vi "Close Panel.vi"(8 "error in (no error)":errorcluster, 10 "Panel":refnum<class "Panel.lvclass">, 11 "Manager in":refnum<class "Manager.lvclass">) -> (0 "error out":errorcluster, 3 "Manager out":refnum<class "Manager.lvclass">)   [LabVIEW 2020, in "OOPanel.lvlib" / "Manager.lvclass"]
uses:
  Manager.lvclass
  Manager.lvclass/Manager.ctl
  Panel/Panel.lvclass
  Panel/Close Reason.ctl
  OOPanel.lvlib
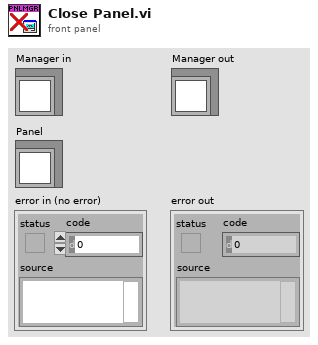
[diagram p1: front panel]
types:
  T1 = typedef "OOPanel.lvlib/Close Reason.ctl" = enum16{"Shutdown", "Close"}
  T2 = typedef "OOPanel.lvlib/Visibility State.ctl" = enum16{"Idle", "Closed", "Hidden", "Visible", "Subpanel"}
  T3 = typedef "OOPanel.lvlib/Manager.lvclass/Ref Data.ctl" = cluster{"SubPanel Map":T4, "Panels":refnum<class "Panel.lvclass">[]}
  T4 = typedef "OOPanel.lvlib/Manager.lvclass/SubPanel Map.ctl" = cluster{"SubPanels":refnum<vi>[], "Panels":refnum<class "Panel.lvclass">[]}
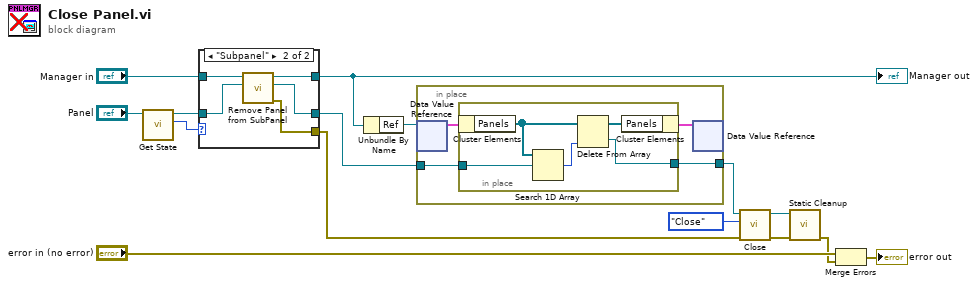
[diagram p0: block diagram]
diagram:
  n1 = call "Get State.vi"("Panel in"="Panel") -> ("State"=w13:T2, "Panel out"=w12:refnum<class "Panel.lvclass">)  [unwired: 8 in, 1 out]
  n2 = case shown="\"Subpanel\"" w13 {
    tunnel: w12 -> [w17 w21]
    tunnel: "Manager in" -> [w16 w22]
    tunnel: [w16 w20] -> w9
    tunnel: [w17 w19] -> w8
    tunnel: [_ w18] -> w7
    frame Default {
    }
    frame "Subpanel" {
      n3 = call "Remove Panel from SubPanel.vi"("Panel In"=w21, "Manager in"=w22) -> ("error out"=w18:errorcluster, "Panel"=w19:refnum<class "Panel.lvclass">, "Manager out"=w20:refnum<class "Manager.lvclass">)  [unwired: 7 in]
    }
  }
  "Manager out" <- w9
  n4 = Unbundle By Name(w9) -> ("Ref"=w10:refnum<data-value>)
  n5 = in-place {
    in-place-border: w8 -> [w24]
    in-place-border: [w23] -> w6
    n6 = in-place-dvr #1(w10) -> (w26:T3)  [unwired: 1 out]
    n7 = in-place {
      in-place-border: w24 -> [w31]
      in-place-border: [w27] -> w23
      n8 = in-place-cluster #2(w26) -> ("Panels"=w30:refnum<class "Panel.lvclass">[])
      n9 = Search 1D Array(1D array=w30, element=w31) -> (index of element=w29:i32)  [unwired: 1 in]
      n10 = Delete From Array(array=w30, index=w29) -> (deleted portion=w27:refnum<class "Panel.lvclass">, array with subset deleted=w28:refnum<class "Panel.lvclass">[])  [unwired: 1 in]
      n11 = in-place-cluster #2("Panels"=w28) -> (w25:T3)
    }
    n12 = in-place-dvr #1(w25) -> ()  [unwired: 2 out]
  }
  n13 = call "Close.vi"("error in (no error)"=w7, "Reason"=Close_Reason."Close", "Panel in"=w6) -> ("error out"=w2:errorcluster, "Panel out"=w3:refnum<class "Panel.lvclass">)  [unwired: 7 in]
  n14 = call "Static Cleanup.vi"("error in (no error)"=w2, "Panel in"=w3) -> ("error out"=w1:errorcluster)  [unwired: 9 in]
  n15 = Merge Errors("error in (no error)", w1) -> (→"error out":errorcluster)
